vi "Close.vi"(8 "error in (no error)":errorcluster, 11 "Ismatech Settings":T1={"VISA resource name"="", "Simulated?"=FALSE, "Pump Number"=1.0, "Reverse?"=FALSE} {"Pump Number" min=1.0 max=20.0 step=1.0}) -> (0 "error out":errorcluster, 3 "Ismatech Settings":T1={"VISA resource name"="", "Simulated?"=FALSE, "Pump Number"=1.0, "Reverse?"=FALSE} {"Pump Number" min=1.0 max=20.0 step=1.0})   [LabVIEW 2018, in "Ismatec ISM 831C.lvlib"]
uses:
  Ismatec ISM 831C.lvlib
  Controls/Ismatech Settings Cluster.ctl
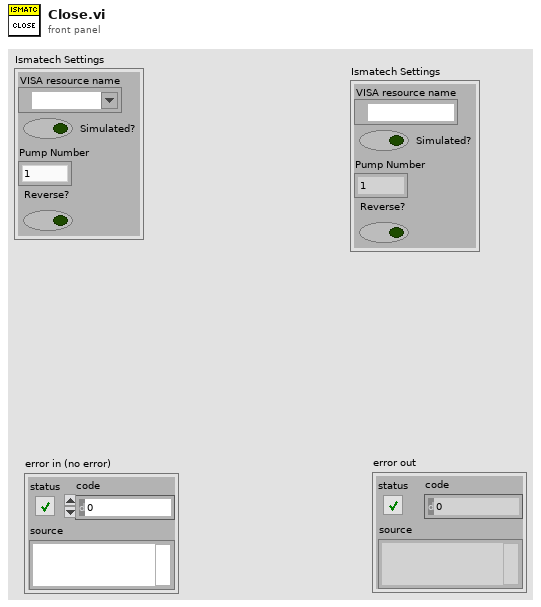
[diagram p1: front panel]
types:
  T1 = typedef "Ismatec ISM 831C.lvlib/Ismatech Settings Cluster.ctl" = cluster{"VISA resource name":refnum<visa-resource-name>, "Simulated?":bool, "Pump Number":dbl, "Reverse?":bool}
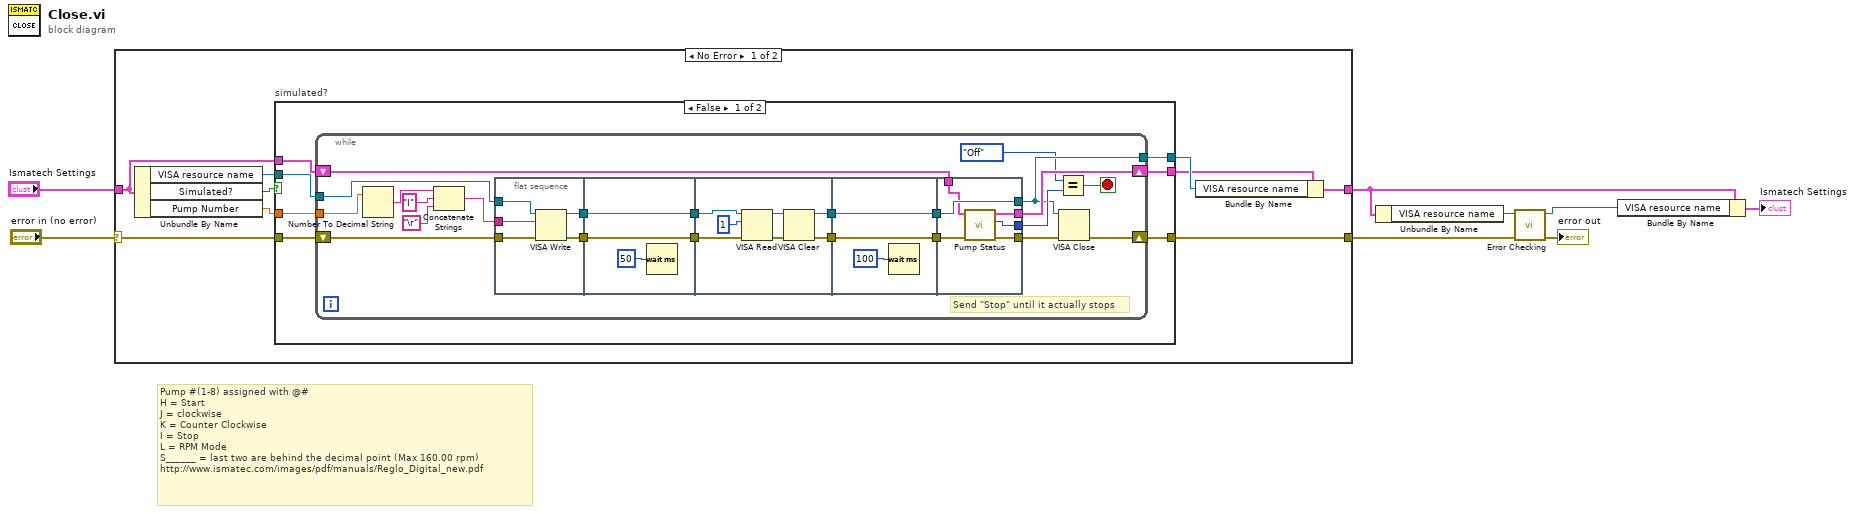
[diagram p0: block diagram]
diagram:
  # "Pump #(1-8) assigned with @#\nH = Start\nJ = clockwise\nK = Counter Clockwise\nI = Stop\nL = RPM Mode\nS______ = last two are behind the decimal point (Max 160.00 rpm)\nhttp://www.ismatec.com/images/pdf/manuals/Reglo_Digital_new.pdf"
  n1 = case shown="No Error" "error in (no error)" {
    selector: "error in (no error)" -> [w12 w76]
    tunnel: [w16 w76] -> w4
    tunnel: [w13 w75] -> w1
    tunnel: "Ismatech Settings" -> [w9 w75]
    frame No Error {
      n2 = Unbundle By Name(w9) -> ("VISA resource name"=w11:refnum<visa-resource-name>, "Simulated?"=w17:bool, "Pump Number"=w14:dbl)
      n3 = case "simulated?" shown="False" w17 {
        tunnel: [w24 w72] -> w16
        tunnel: [w18 w73] -> w15
        tunnel: w14 -> [w23 _]
        tunnel: w12 -> [w22 w72]
        tunnel: w11 -> [w21 w73]
        tunnel: w9 -> [w20 w74]
        tunnel: [w19 w74] -> w10
        frame False {
          n4 = while {
            tunnel: w23 -> [w35]
            tunnel: w21 -> [w31]
            shift-right: [w39] -> w24
            shift-left: w22 -> [w33]
            shift-right: [w29] -> w19
            shift-left: w20 -> [w30]
            tunnel: [w26] -> w18
            stop <- w28 stop-if-true
            # "Send \"Stop\" until it actually stops"
            n5 = Number To Decimal String(number=w35) -> (decimal integer string=w34:string)  [unwired: 1 in]
            n6 = Concatenate Strings(w34, "I" ("string"), "\r") -> (w32:string)
            n7 = flat-sequence {
              tunnel: w33 -> [w52]
              tunnel: w32 -> [w51]
              tunnel: w31 -> [w50]
              tunnel: [w49] -> w47
              tunnel: [w48] -> w46
              tunnel: [w54] -> w45
              tunnel: w47 -> [w54]
              tunnel: w46 -> [w53]
              tunnel: [w53] -> w44
              tunnel: w45 -> [w57]
              tunnel: w44 -> [w56]
              tunnel: [w59] -> w43
              tunnel: [w58] -> w42
              tunnel: w43 -> [w65]
              tunnel: w42 -> [w64]
              tunnel: [w65] -> w41
              tunnel: [w64] -> w40
              tunnel: [w69] -> w36
              tunnel: [w71] -> w26
              tunnel: w41 -> [w71]
              tunnel: w40 -> [w70]
              tunnel: w30 -> [w68]
              tunnel: [w67] -> w29
              tunnel: [w66] -> w27
              frame #0 {
                n8 = VISA Write(VISA resource name=w50, write buffer=w51, error in (no error)=w52) -> (VISA resource name out=w49:refnum<visa-resource-name>, error out=w48:errorcluster)  [unwired: 1 out]
              }
              frame #1 {
                n9 = Wait (ms)(milliseconds to wait=u32 50) -> ()  [unwired: 1 out]
              }
              frame #2 {
                n10 = VISA Read(VISA resource name=w57, byte count=u32 1, error in (no error)=w56) -> (VISA resource name out=w61:refnum<visa-resource-name>, error out=w62:errorcluster)  [unwired: 2 out]
                n11 = VISA Clear(VISA resource name=w61, error in (no error)=w62) -> (VISA resource name out=w59:refnum<visa-resource-name>, error out=w58:errorcluster)
              }
              frame #3 {
                n12 = Wait (ms)(milliseconds to wait=u32 100) -> ()  [unwired: 1 out]
              }
              frame #4 {
                n13 = call "Pump Status.vi"("error in (no error)"=w70, "Ismatech Settings"=w68) -> ("error out"=w69:errorcluster, "Pump On?"=w66:enum16{"Off", "On", "Not Initialized"}, "Ismatech Settings"=w67:T1)  [unwired: 6 in, 1 out]
              }
            }
            n14 = Equal?(x=enum16{"Off", "On", "Not Initialized"}."Off", y=w27) -> (x = y?=w28:bool)
            n15 = VISA Close(VISA resource name=w26, error in (no error)=w36) -> (error out=w39:errorcluster)
          }
        }
        frame True {
        }
      }
      n16 = Bundle By Name(cluster=w10, "VISA resource name"=w15) -> (w13:T1)
    }
    frame Error {
    }
  }
  n17 = Unbundle By Name(w1) -> ("VISA resource name"=w6:refnum<visa-resource-name>)
  n18 = call "Error Checking.vi"("error in (no error)"=w4, "VISA resource name"=w6) -> ("error out"=→"error out":errorcluster, "VISA resource name"=w5:refnum<visa-resource-name>)  [unwired: 7 in, 1 out]
  n19 = Bundle By Name(cluster=w1, "VISA resource name"=w5) -> (→"Ismatech Settings":T1)
